vi "FPGA_speed_control.vi"() -> ()   [LabVIEW 2018]
uses:
  <vilib>/Platform/TimedLoop/XDataNode/timing_clust.ctl
  <vilib>/Platform/TimedLoop/XDataNode/nitl_modes.ctl
  <vilib>/Platform/TimedLoop/XDataNode/wakeup.ctl
  <vilib>/rvi/Emulation/niFpgaGetClockAttributes.vi
  <vilib>/rvi/Emulation/niFpgaSctlEmulationGetInTimedLoop.vi
  <vilib>/rvi/Emulation/niFpgaEmulationReportErrorSimple.vi
  <vilib>/rvi/eio/common/nirviEmuTemplateMethod_errors.vi
  <vilib>/rvi/Emulation/niFpgaCriticalErrorInLSC.vi
  <vilib>/rvi/Emulation/niFpgaProcessEmulError.vi
  <vilib>/eio/EIONode/EIONode.xnode
  <vilib>/platform/TimedLoop/XDataNode/XDataNode.xnode
  <vilib>/Platform/TimedLoop/XDataNode/XDNodeRunTimeDep.lvlib
panel:
  in  "pwm_freq":u32=1000
  in  "speed_step":u32
  out "speed":i16
  in  "pos_update_us":u32=10
  out "coerced(x)":u32
  out "speed up":bool
  out "speed chart":i16(graph)
  in  "ai_delayus":u32=10
  in  "sp_min_limit":u16=400
  in  "sp_max_limit":u16=600
  in  "speed_sp":i16=40
  in  "delay_pwm_us":u32=100
  out "AI0":u16=1344
  out "dAI":i16=8
  out "dt_pwm_ms":u32=300 caption="Count(uSec)"
  out "busy":bool
  in  "dt_m_us":u32=1 caption="delay_M_ms"
  in  "setpt":i16
  out "backward":bool
  out "pos":i16=1241
  out "err cnt":i16
  in  "reset":bool
  out "off_track":bool
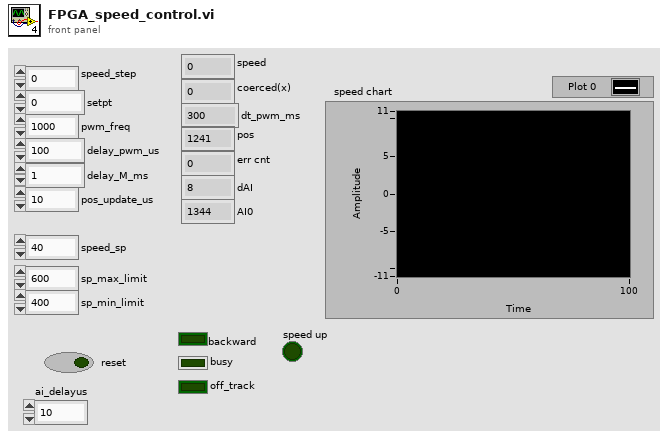
[diagram p1: front panel]
types:
  T1 = typedef "XDNodeRunTimeDep.lvlib/timing_clust.ctl" = cluster{"Expected End [f-1]":u64, "Actual End [f-1]":u64, "Finished Late? [f-1]":bool, "Expected End [i-1]":u64, "Actual End [i-1]":u64, "Finished Late? [i-1]":bool, "Expected Start [i]":u64, "Actual Start [i]":u64, "Expected Start [f]":u64, "Actual Start [f]":u64, "Source Name":string, "Structure Name":string, "Period":i64, "Deadline":i64, "Offset":i64, "Start":i64, "Priority":i32, "Timeout":i32, "Mode":T2, "Wakeup Reason":T3, "Error":errorcluster, "Source Type":string, "Secondary Source Type":string, "Global End Time":u64, "Global Start Time":u64, "Frame Duration":u64, "Iteration Duration":u64, "Assigned CPU":i32, "I/O Scan Engine Mode":u32}
  T2 = typedef "XDNodeRunTimeDep.lvlib/nitl_modes.ctl" = enum32{"No Change", "Process missed periods, maintain original phase", "Discard missed periods, maintain original phase", "Process missed periods, ignore original phase", "Discard missed periods, ignore original phase"}
  T3 = typedef "XDNodeRunTimeDep.lvlib/wakeup.ctl" = enum32{"Normal", "Aborted", "Asynchronous wakeup", "Timing source error", "Timed loop error", "Timeout"}
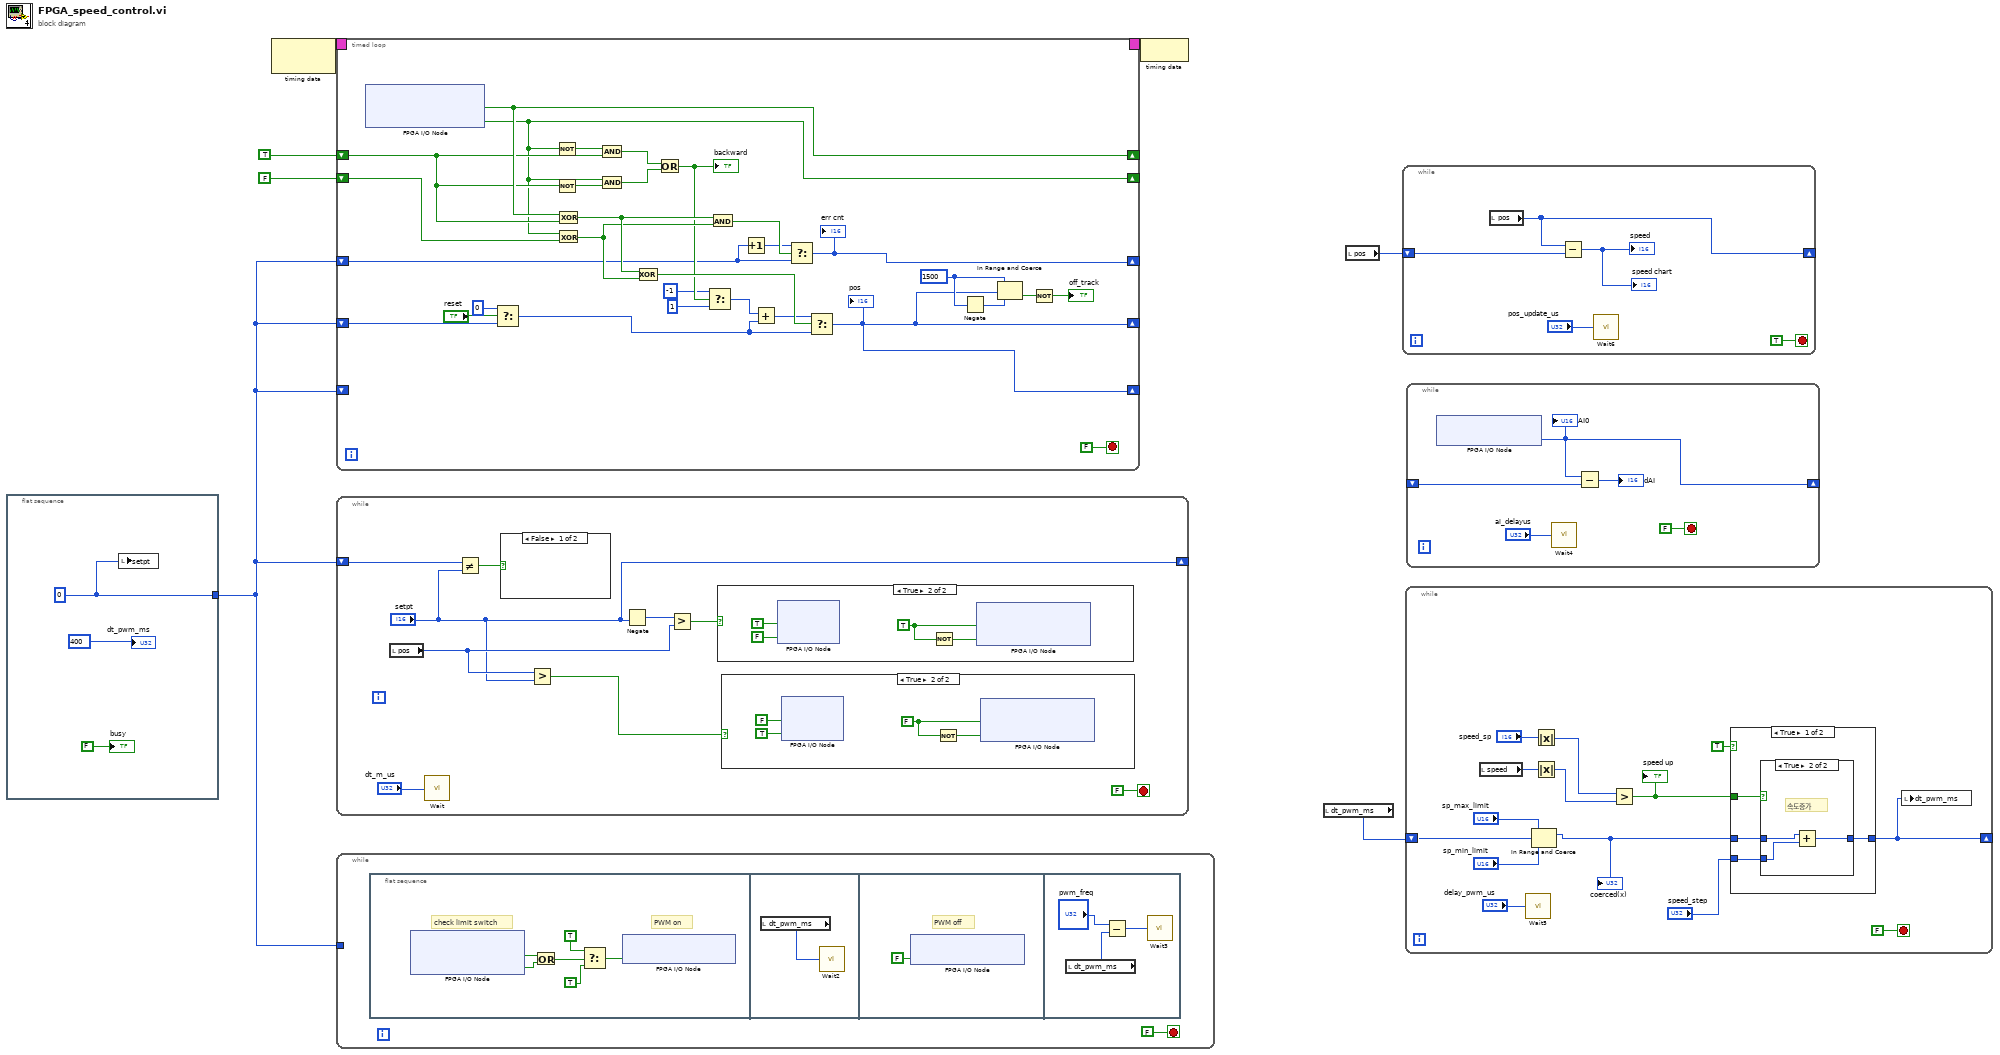
[diagram p0: block diagram]
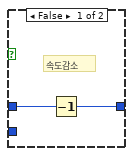
[diagram p2: hidden frame]
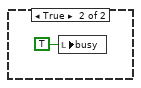
[diagram p5: hidden frame]
diagram:
  n1 = flat-sequence {
    tunnel: [w9] -> w2
    frame #0 {
      w9 = i16 0
      n2 = local write "setpt"(w9) -> ()
      "busy" <- FALSE ("status")
      "dt_pwm_ms" <- u32 400 ("dt_pwm_ms")
    }
  }
  n3 = node-c288() -> (w7:T1)  [unwired: 1 in]
  n4 = timed-loop {
    timing: w7 -> [_]
    timing-out: [_] -> w6
    shift-right: [w35] -> _
    shift-left: TRUE ("ConnectorA/DIO11") -> [w34]
    shift-right: [w33] -> _
    shift-left: FALSE ("ConnectorA/DIO12") -> [w32]
    shift-right: [w11] -> _
    shift-left: w2 -> [w18]
    shift-right: [w20] -> _
    shift-left: w2 -> [w21]
    shift-right: [w11] -> _
    shift-left: w2 -> [_]
    stop <- FALSE stop-if-true
    w12 = i16 1500 ("upper limit")
    n5 = xnode "FPGA I/O Node"() -> ("ConnectorA/DIO11"=w35:bool, "ConnectorA/DIO12"=w33:bool)  [unwired: 2 in, 2 out]
    n6 = Select(t=i16 0, s="reset", f=w18) -> (s? t:f=w16:i16)
    n7 = Not(x=w33) -> (.not. x?=w39:bool)
    n8 = Not(x=w34) -> (.not. x?=w38:bool)
    n9 = Exclusive Or(1:w34, 2:w35) -> (0:w31:bool)
    n10 = Exclusive Or(1:w32, 2:w33) -> (0:w30:bool)
    n11 = And(x=w39, y=w34) -> (x .and. y?=w36:bool)
    n12 = And(x=w33, y=w38) -> (x .and. y?=w37:bool)
    n13 = Exclusive Or(1:w30, 2:w31) -> (0:w29:bool)
    n14 = Or(x=w36, y=w37) -> (x .or. y?=w28:bool)
    "backward" <- w28
    n15 = Select(t=i16 -1, s=w28, f=i16 1) -> (s? t:f=w25:i16)
    n16 = And(x=w31, y=w30) -> (x .and. y?=w23:bool)
    n17 = Increment(x=w21) -> (x+1=w22:i16)
    n18 = Add(x=w25, y=w16) -> (x+y=w24:i16)
    n19 = Select(t=w22, s=w23, f=w21) -> (s? t:f=w20:i16)
    "err cnt" <- w20
    n20 = Select(t=w24, s=w29, f=w16) -> (s? t:f=w11:i16)
    "pos" <- w11
    n21 = Negate(x=w12) -> (-x=w13:i16)
    n22 = In Range and Coerce(upper limit=w12, x=w11, lower limit=w13) -> (In Range?=w15:bool)  [unwired: 1 out]
    n23 = Not(x=w15) -> (.not. x?=→"off_track":bool)
  }
  n24 = while {
    shift-right: ["setpt"] -> _
    shift-left: w2 -> [w49]
    stop <- FALSE stop-if-true
    n25 = local read "pos"() -> (w45:i16)
    n26 = call "Wait"("Count(uSec)"="dt_m_us") -> ()  [unwired: 1 out]
    n27 = Not Equal?(x=w49, y="setpt") -> (x != y?=w48:bool)
    n28 = case shown="False" w48 {
      frame False {
      }
      frame True {
        n29 = local write "busy"(TRUE ("busy")) -> ()
      }
    }
    n30 = Greater?(x=w45, y="setpt") -> (0:w43:bool)
    n31 = Negate(x="setpt") -> (-x=w47:i16)
    n32 = Greater?(x=w47, y=w45) -> (0:w46:bool)
    n33 = case shown="True" w46 {
      frame False {
      }
      frame True {
        w52 = TRUE ("dir")
        n34 = xnode "FPGA I/O Node"("LED0"=TRUE, "LED1"=FALSE) -> ()  [unwired: 2 in, 2 out]
        n35 = Not(x=w52) -> (.not. x?=w55:bool)
        n36 = xnode "FPGA I/O Node"("ConnectorA/DIO6"=w52, "ConnectorA/DIO5"=w55) -> ()  [unwired: 2 in, 2 out]
      }
    }
    n37 = case shown="True" w43 {
      frame False {
      }
      frame True {
        w57 = FALSE ("dir")
        n38 = xnode "FPGA I/O Node"("LED0"=FALSE, "LED1"=TRUE) -> ()  [unwired: 2 in, 2 out]
        n39 = Not(x=w57) -> (.not. x?=w60:bool)
        n40 = xnode "FPGA I/O Node"("ConnectorA/DIO6"=w57, "ConnectorA/DIO5"=w60) -> ()  [unwired: 2 in, 2 out]
      }
    }
  }
  n41 = while {
    tunnel: w2 -> [_]
    stop <- FALSE stop-if-true
    n42 = flat-sequence {
      frame #0 {
        # "check limit switch"
        # "PWM on"
        n43 = xnode "FPGA I/O Node"() -> ("ConnectorA/DIO0"=w66:bool, "ConnectorA/DIO1"=w67:bool)  [unwired: 2 in, 2 out]
        n44 = Or(x=w66, y=w67) -> (x .or. y?=w65:bool)
        n45 = Select(t=TRUE, s=w65, f=TRUE ("ConnectorA/DIO8")) -> (s? t:f=w64:bool)
        n46 = xnode "FPGA I/O Node"("ConnectorA/DIO8"=w64) -> ()  [unwired: 1 in, 1 out]
      }
      frame #1 {
        n47 = local read "dt_pwm_ms"() -> (w68:u32)
        n48 = call "Wait2"("Count(uSec)"=w68) -> ()  [unwired: 1 out]
      }
      frame #2 {
        # "PWM off"
        n49 = xnode "FPGA I/O Node"("ConnectorA/DIO8"=FALSE) -> ()  [unwired: 1 in, 1 out]
      }
      frame #3 {
        n50 = local read "dt_pwm_ms"() -> (w72:u32)
        n51 = Subtract(x="pwm_freq", y=w72) -> (x-y=w70:u32)
        n52 = call "Wait3"("Count(uSec)"=w70) -> ()  [unwired: 1 out]
      }
    }
  }
  n53 = node-c288(w6) -> ()
  n54 = local read "dt_pwm_ms"() -> (w3:u32)
  n55 = local read "pos"() -> (w1:i16)
  n56 = while {
    shift-right: [w75] -> _
    shift-left: w1 -> [w74]
    stop <- TRUE stop-if-true
    n57 = local read "pos"() -> (w75:i16)
    n58 = Subtract(x=w75, y=w74) -> (x-y=→"speed" →"speed chart":i16)
    n59 = call "Wait6"("Count(uSec)"="pos_update_us") -> ()  [unwired: 1 out]
  }
  n60 = while {
    shift-right: [w89] -> _
    shift-left: w3 -> [w88]
    stop <- FALSE stop-if-true
    n61 = local read "speed"() -> (w79:i16)
    n62 = call "Wait5"("Count(uSec)"="delay_pwm_us") -> ()  [unwired: 1 out]
    n63 = In Range and Coerce(upper limit="sp_max_limit", x=w88, lower limit="sp_min_limit") -> (coerced(x)=w85:u32)  [unwired: 1 out]
    "coerced(x)" <- w85
    n64 = Absolute Value(x="speed_sp") -> (abs(x)=w82:i16)
    n65 = Absolute Value(x=w79) -> (abs(x)=w81:i16)
    n66 = Greater?(x=w82, y=w81) -> (0:w83:bool)
    "speed up" <- w83
    n67 = case shown="True" TRUE {
      tunnel: [w95 w101] -> w89
      tunnel: w85 -> [w94 w101]
      tunnel: w83 -> [w93 _]
      tunnel: "speed_step" -> [w92 _]
      frame True {
        n68 = case shown="True" w93 {
          tunnel: w94 -> [w97 w99]
          tunnel: [w96 w100] -> w95
          tunnel: w92 -> [_ w98]
          frame False {
            # "속도감소"
            n69 = Decrement(x=w97) -> (x-1=w96:u32)
          }
          frame True {
            # "속도증가"
            n70 = Add(x=w99, y=w98) -> (x+y=w100:u32)
          }
        }
      }
      frame False {
      }
    }
    n71 = local write "dt_pwm_ms"(w89) -> ()
  }
  n72 = while {
    shift-right: [w102] -> _
    shift-left: _ -> [w103]
    stop <- FALSE stop-if-true
    n73 = xnode "FPGA I/O Node"() -> ("ConnectorA/AI0"=w102:u16)  [unwired: 1 in, 1 out]
    "AI0" <- w102
    n74 = call "Wait4"("Count(uSec)"="ai_delayus") -> ()  [unwired: 1 out]
    n75 = Subtract(x=w102, y=w103) -> (x-y=→"dAI":u16)
  }
